vi "IDS_system_resetError.vi"(8 "error in (no error)":errorcluster, 10 "performRenormalisation":bool, 11 "deviceHandle":i32) -> (0 "error out":errorcluster, 3 "deviceHandle out":i32)   [LabVIEW 2016]
doc: "int IDS_DLL IDS_system_resetError();"
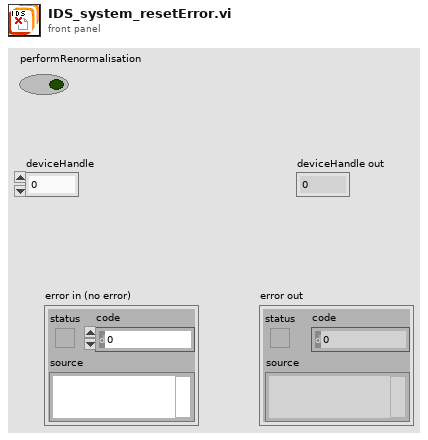
[diagram p1: front panel]
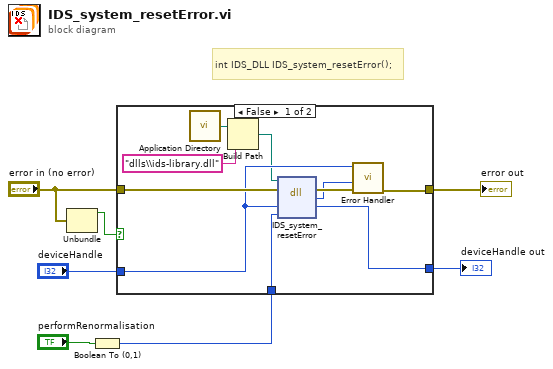
[diagram p0: block diagram]
diagram:
  # "int IDS_DLL IDS_system_resetError();"
  n1 = Unbundle("error in (no error)") -> ("status"=w3:bool)  [unwired: 2 out]
  n2 = Boolean To (0,1)(Boolean="performRenormalisation") -> (0, 1=w1:i16)
  n3 = case shown="False" w3 {
    tunnel: "error in (no error)" -> [w17 w19]
    tunnel: [w15 w19] -> w7
    tunnel: "deviceHandle" -> [w12 w18]
    tunnel: [w14 w18] -> w5
    tunnel: w1 -> [w11 _]
    frame False {
      n4 = call <vilib>:"Application Directory.vi"() -> ("Application Directory"=w10:path)
      n5 = Build Path(base path=w10, name or relative path="dlls\\ids-library.dll" ("ipAddress")) -> (appended path=w8:path)
      n6 = dll-call lib="C:/Users/matheus/Desktop/LabVIEW_Draft_V1.6.0/dlls/ids-library.*" fn="IDS_system_resetError"(path in=w8, error in=w17, "deviceHandle"=w12, "performRenormalization"=w11) -> (error out=w16:errorcluster, "return type"=w13:i32, "deviceHandle"=w14:i32)  [unwired: 2 in, 1 out]
      n7 = call "Error Handler.vi"("error in (no error)"=w16, "error code"=w13, "deviceHandle"=w12) -> ("error out"=w15:errorcluster)  [unwired: 7 in, 1 out]
    }
    frame True {
    }
  }
  "error out" <- w7
  "deviceHandle out" <- w5
